vi "ReferencedVariables_ReadWriteReferencedVariable_4x4x4.vi"(8 "error in (no error)":errorcluster, 10 "ReplaceWithtypeDef":dbl, 11 "reference in":refnum<class>) -> (0 "error out":errorcluster, 3 "reference out":refnum<class>)   [LabVIEW 2010]
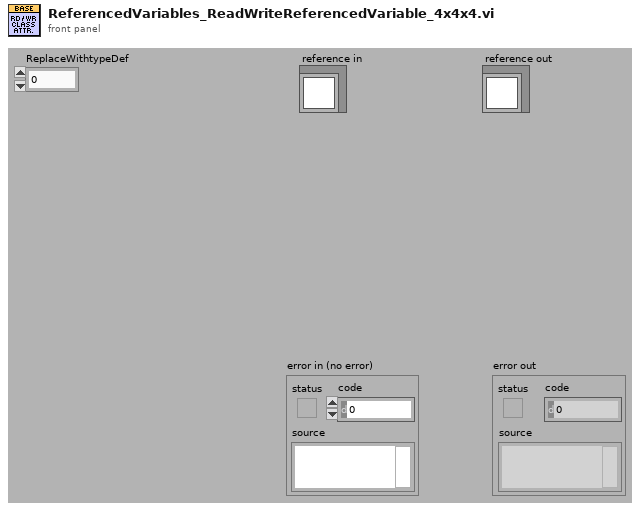
[diagram p1: front panel]
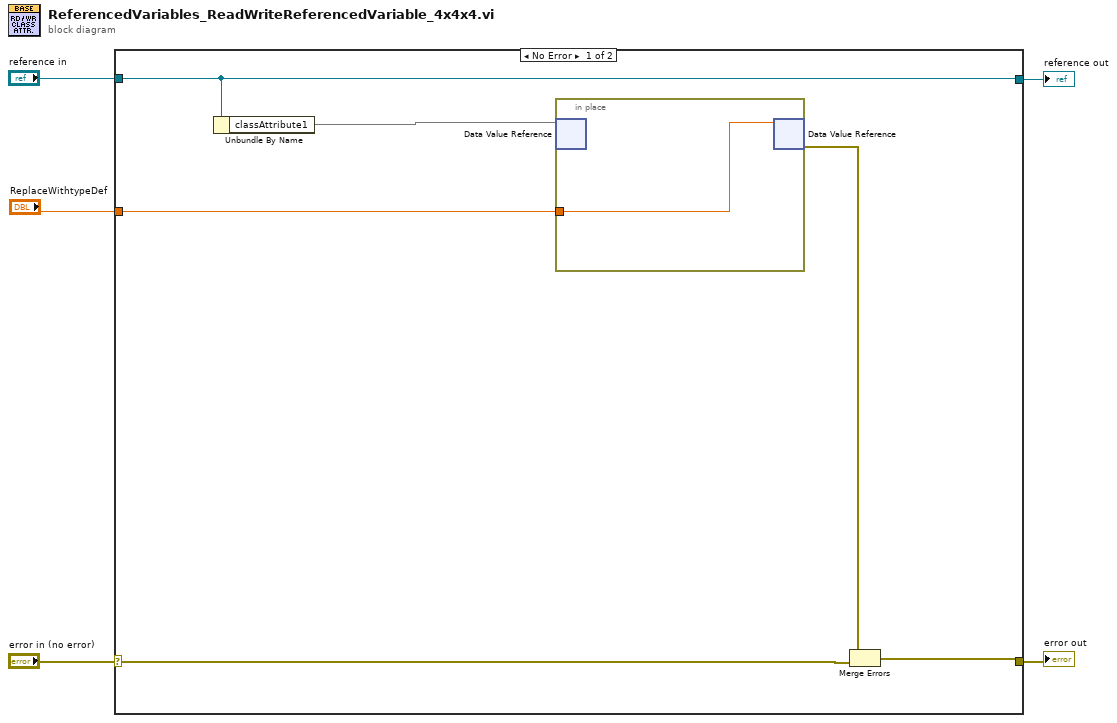
[diagram p0: block diagram]
diagram:
  n1 = case shown="No Error" "error in (no error)" {
    selector: "error in (no error)" -> [w8 w14]
    tunnel: [w11 w14] -> w4
    tunnel: [w6 w13] -> w2
    tunnel: "reference in" -> [w6 w13]
    tunnel: "ReplaceWithtypeDef" -> [w7 _]
    frame No Error {
      n2 = Unbundle By Name(w6) -> ("classAttribute1"=w10)
      n3 = in-place {
        in-place-border: w7 -> [w12]
        n4 = in-place-dvr #1(w10) -> ()  [unwired: 2 out]
        n5 = in-place-dvr #1(w12) -> (w9:errorcluster)  [unwired: 1 out]
      }
      n6 = Merge Errors(w9, w8) -> (w11:errorcluster)
    }
    frame Error {
    }
  }
  "error out" <- w4
  "reference out" <- w2
